vi "Initialize ProgressBar.vi"(8 "error in (no error)":errorcluster, 9 "Scale Min":dbl format="%#_13g", 10 "Scale Max":dbl=10.0 format="%#_13g", 11 "ProgressBar in":refnum<class "ProgressBar.lvclass">) -> (0 "error out":errorcluster, 3 "ProgressBar out":refnum<class "ProgressBar.lvclass">)   [LabVIEW 2019, in "ProgressBar.lvclass"]
uses:
  ProgressBar.lvclass
  <vilib>/JKI/JKI SMO/SMO/SMO.lvclass
  C:/Program Files (x86)/National Instruments/LabVIEW 2019/vi.lib/JKI/JKI SMO/SMO.UI/SMO.UI.lvclass
  C:/Program Files (x86)/National Instruments/LabVIEW 2019/vi.lib/JKI/JKI SMO/SMO/SMO.lvclass
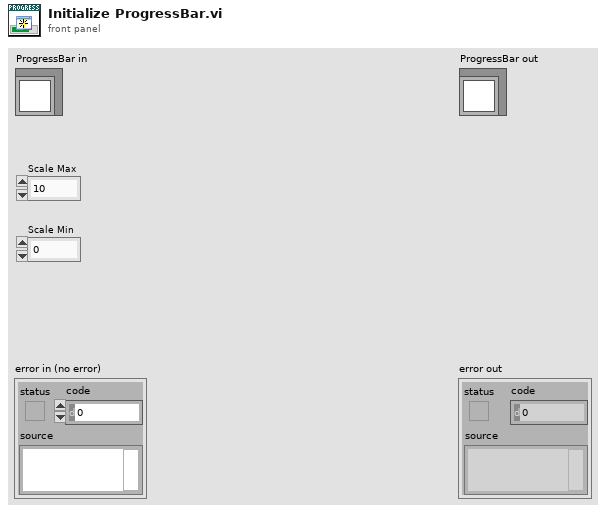
[diagram p1: front panel]
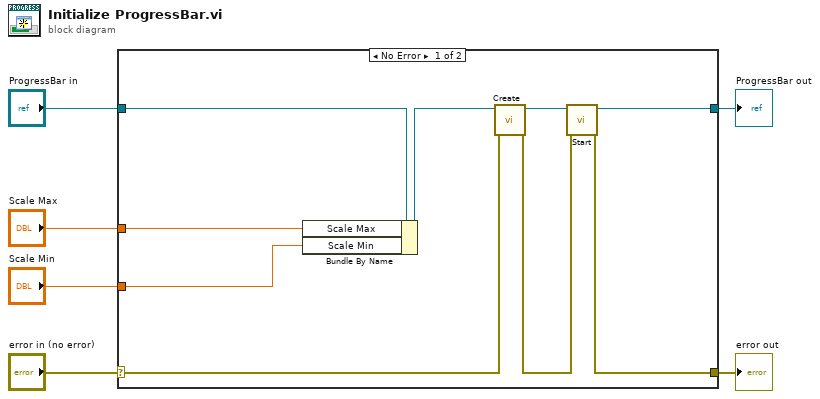
[diagram p0: block diagram]
diagram:
  n1 = case shown="No Error" "error in (no error)" {
    selector: "error in (no error)" -> [w12 w17]
    tunnel: [w10 w17] -> w5
    tunnel: [w8 w16] -> w3
    tunnel: "ProgressBar in" -> [w7 w16]
    tunnel: "Scale Max" -> [w14 _]
    tunnel: "Scale Min" -> [w13 _]
    frame No Error {
      n2 = Bundle By Name(cluster=w7, "Scale Max"=w14, "Scale Min"=w13) -> (w15:refnum<class "ProgressBar.lvclass">)
      n3 = call <vilib>:"Create.vi"("error in (no error)"=w12, "SMO"=w15) -> ("error out"=w11:errorcluster, "SMO out"=w9:refnum<class "ProgressBar.lvclass">)  [unwired: 7 in, 1 out]
      n4 = call <vilib>:"Start.vi"("error in (no error)"=w11, "SMO"=w9) -> ("error out"=w10:errorcluster, "SMO out"=w8:refnum<class "ProgressBar.lvclass">)  [unwired: 8 in]
    }
    frame Error {
    }
  }
  "error out" <- w5
  "ProgressBar out" <- w3
